vi "Factorial of a number.vi"() -> ()   [LabVIEW 2020]
panel:
  out "Factorial":dbl
  in  "Input Number":dbl
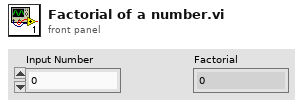
[diagram p1: front panel]
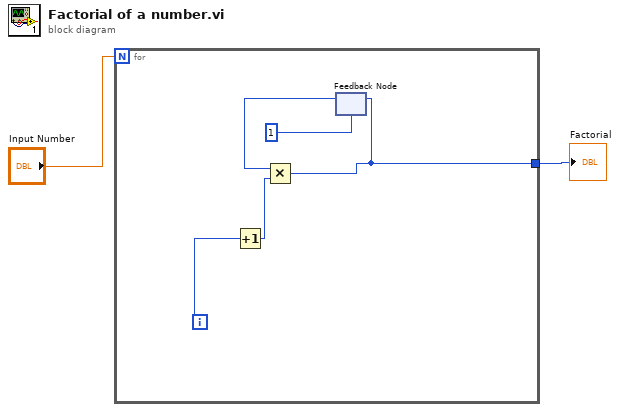
[diagram p0: block diagram]
diagram:
  n1 = for {
    N: "Input Number" -> [_]
    tunnel: [w3] -> w1
    i -> [w7]
    n2 = Increment(x=w7) -> (x+1=w6:i32)
    n3 = feedback #1(1) -> (w5:i32)
    n4 = Multiply(x=w5, y=w6) -> (x*y=w3:i32)
    n5 = feedback-in #1(w3) -> ()
  }
  "Factorial" <- w1
